vi "CreateGroup.vi"(6 "ChanGroups":refnum<class "ChanGrp.lvclass">[](array[class]), 7 "Modbus URL":string, 8 "error in":errorcluster, 10 "ReadBlk":i32, 11 "Rate":dbl) -> (0 "error out":errorcluster, 3 "Timing Group":refnum<class "TimingGrp.lvclass">)   [LabVIEW 2012, in "Configuration Grandmaster.lvlib" / "TimingGrp.lvclass"]
uses:
  TimingGrp.lvclass
  Class Chan Group/ChanGrp.lvclass
  TimingGrp.lvclass/TimingGrp.ctl
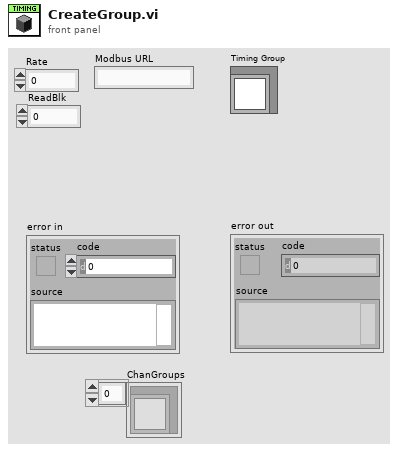
[diagram p1: front panel]
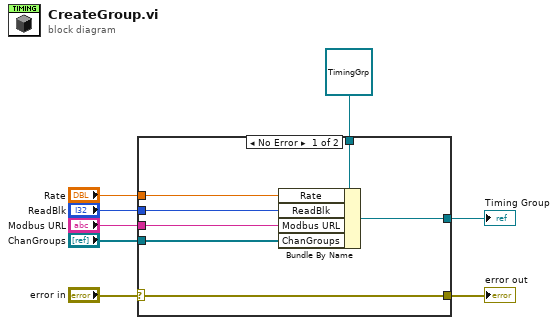
[diagram p0: block diagram]
diagram:
  n1 = case shown="No Error" "error in" {
    selector: "error in" -> [w11 w16]
    tunnel: refnum<class "TimingGrp.lvclass"> refnum ("TimingGrp.lvclass") -> [w15 w17]
    tunnel: "Rate" -> [w14 _]
    tunnel: "ReadBlk" -> [w13 _]
    tunnel: [w12 w17] -> w5
    tunnel: [w11 w16] -> w3
    tunnel: "Modbus URL" -> [w10 _]
    tunnel: "ChanGroups" -> [w9 _]
    frame No Error {
      n2 = Bundle By Name(cluster=w15, "Rate"=w14, "ReadBlk"=w13, "Modbus URL"=w10, "ChanGroups"=w9) -> (w12:refnum<class "TimingGrp.lvclass">)
    }
    frame Error {
    }
  }
  "Timing Group" <- w5
  "error out" <- w3
